vi "上位机.vi"() -> ()   [LabVIEW 2017]
uses:
  HslCommunication.dll
panel:
  in  "启动时读取数据":bool
  out "总时间 2":u32 format="%.0fms"
  out "PLC单次读写时间":u32 format="%.0fms"
  out "数值":i32
  out "Q14.6 备用":bool
  out "Q10.0 三色灯红":bool
  out "Q10.1 三色灯黄":bool
  out "Q10.2 三色灯绿":bool
  out "Q10.6 循环停止指示":bool
  out "Q10.7 原点指示":bool
  out "Q11.0 备用":bool
  out "Q14.0 工位1选择检测型腔":bool
  out "Q14.1 工位1选择检测水道":bool
  out "Q14.2 工位1选择检测回油道":bool
  out "Q14.7 辊道电机变频器启动":bool
  out "Q15.0 试漏启动":bool
  out "Q15.1 试漏频道0#":bool
  out "Q15.2 试漏频道1#":bool
  out "Q15.3 试漏频道2#":bool
  out "Q15.4 试漏频道3#":bool
  out "Q15.5 备用":bool
  out "Q15.6 备用":bool
  out "Q15.7 备用":bool
  out "Q14.3 工位1型腔泄压":bool
  out "Q14.4 工位1水道泄压":bool
  out "Q14.5 工位1选择回油道泄压":bool
  out "Q10.3 三色灯蜂鸣":bool
  out "Q10.4 故障复位指示":bool
  out "Q10.5 循环启动指示":bool
  out "Q11.1 备用":bool
  out "I10.0 机器人电源反馈":bool
  out "I10.1 伺服电源反馈":bool
  out "I10.2 输送电源反馈":bool
  out "I10.3 备用":bool
  out "I10.4 备用":bool
  out "I10.5 备用":bool
  out "I10.6 备用":bool
  out "I10.7 备用":bool
  out "I11.0 系统上电":bool
  out "I11.1 急停":bool
  out "I11.2 故障复位":bool
  out "I11.3 备用":bool
  out "I11.4 备用":bool
  out "I12.0 1#萃盘物料上升检测":bool
  out "I12.2 1#萃盘上料皮带检测1":bool
  out "I12.4 1#萃盘下料皮带检测1":bool
  out "I12.6 备用":bool
  out "I12.7 备用":bool
  out "I13.0 2#萃盘物料上升检测":bool
  out "I13.1 2#萃盘物料倾斜检测":bool
  out "I13.2 2#萃盘上料皮带检测1":bool
  out "I13.3 2#萃盘上料皮带检测2":bool
  out "I13.4 2#萃盘下料皮带检测1":bool
  out "I13.5 2#萃盘下料皮带检测2":bool
  out "I13.6 备用":bool
  out "I13.7 备用":bool
  out "I14.0 1#X轴气缸原位":bool
  out "I14.1 1#X轴气缸工作位":bool
  out "I14.2 1#Z轴气缸原位":bool
  out "I14.3  1#Z轴气缸工作位":bool
  out "I14.4  2#X轴气缸原位":bool
  out "I14.5  2#X轴气缸工作位":bool
  out "I14.6  2#Z轴气缸原位":bool
  out "I14.7  2#Z轴气缸工作位":bool
  out "I15.0  热熔升降原位":bool
  out "I15.1  热熔升降工作位":bool
  out "I15.2  烧录升降原位":bool
  out "I15.3  烧录升降工作位":bool
  out "I15.4  备用":bool
  out "I15.5  备用":bool
  out "I15.6  备用":bool
  out "I15.7  备用":bool
  out "I12.1 1#萃盘物料倾斜检测":bool
  out "I12.3 1#萃盘上料皮带检测2":bool
  out "I12.5 1#萃盘下料皮带检测2":bool
  in  "缩回按钮":bool
  in  "伸出按钮":bool
  in  "缩回按钮 2":bool
  in  "伸出按钮 2":bool
  in  "缩回按钮 3":bool
  in  "伸出按钮 3":bool
  in  "缩回按钮 4":bool
  in  "伸出按钮 4":bool
  in  "缩回按钮 5":bool
  in  "伸出按钮 5":bool
  in  "缩回按钮 6":bool
  in  "伸出按钮 6":bool
  in  "缩回按钮 7":bool
  in  "伸出按钮 7":bool
  in  "缩回按钮 8":bool
  in  "伸出按钮 8":bool
  in  "缩回按钮 9":bool
  in  "伸出按钮 9":bool
  in  "缩回按钮 10":bool
  in  "伸出按钮 10":bool
  in  "缩回按钮 11":bool
  in  "伸出按钮 11":bool
  in  "缩回按钮 12":bool
  in  "伸出按钮 12":bool
  out "M210.0 自动模式":bool
  out "通讯状态":bool
  out "模式选择":i32(ring) items=["单机模式", "联机模式"]
  out "产品信号":i32(ring) items=["CS-18", ""]
  out "设备状态":i32(ring) items=["准备OK"]
  out "当前报警代码":i32 format="%x"
  out "当前故障代码":i32 format="%x"
  out "1轴转速":dbl
  out "1轴转速 2":dbl
  out "1轴转速 3":dbl
  in  "1#轴位置5":dbl
  in  "1#轴位置3":dbl
  in  "1#轴位置4":dbl
  in  "1#轴位置1":dbl
  in  "1#轴位置2":dbl
  in  "2#轴位置5":dbl
  in  "2#轴位置3":dbl
  in  "2#轴位置4":dbl
  in  "2#轴位置1":dbl
  in  "2#轴位置2":dbl
  out "连接成功 2":bool
  # "IO布尔读取DB1.4"
  # "布尔写入DB1.0"
  # "IO布尔读取DB1.20"
  # "浮点数写入DB1.284"
  # "浮点数读取DB1.160"
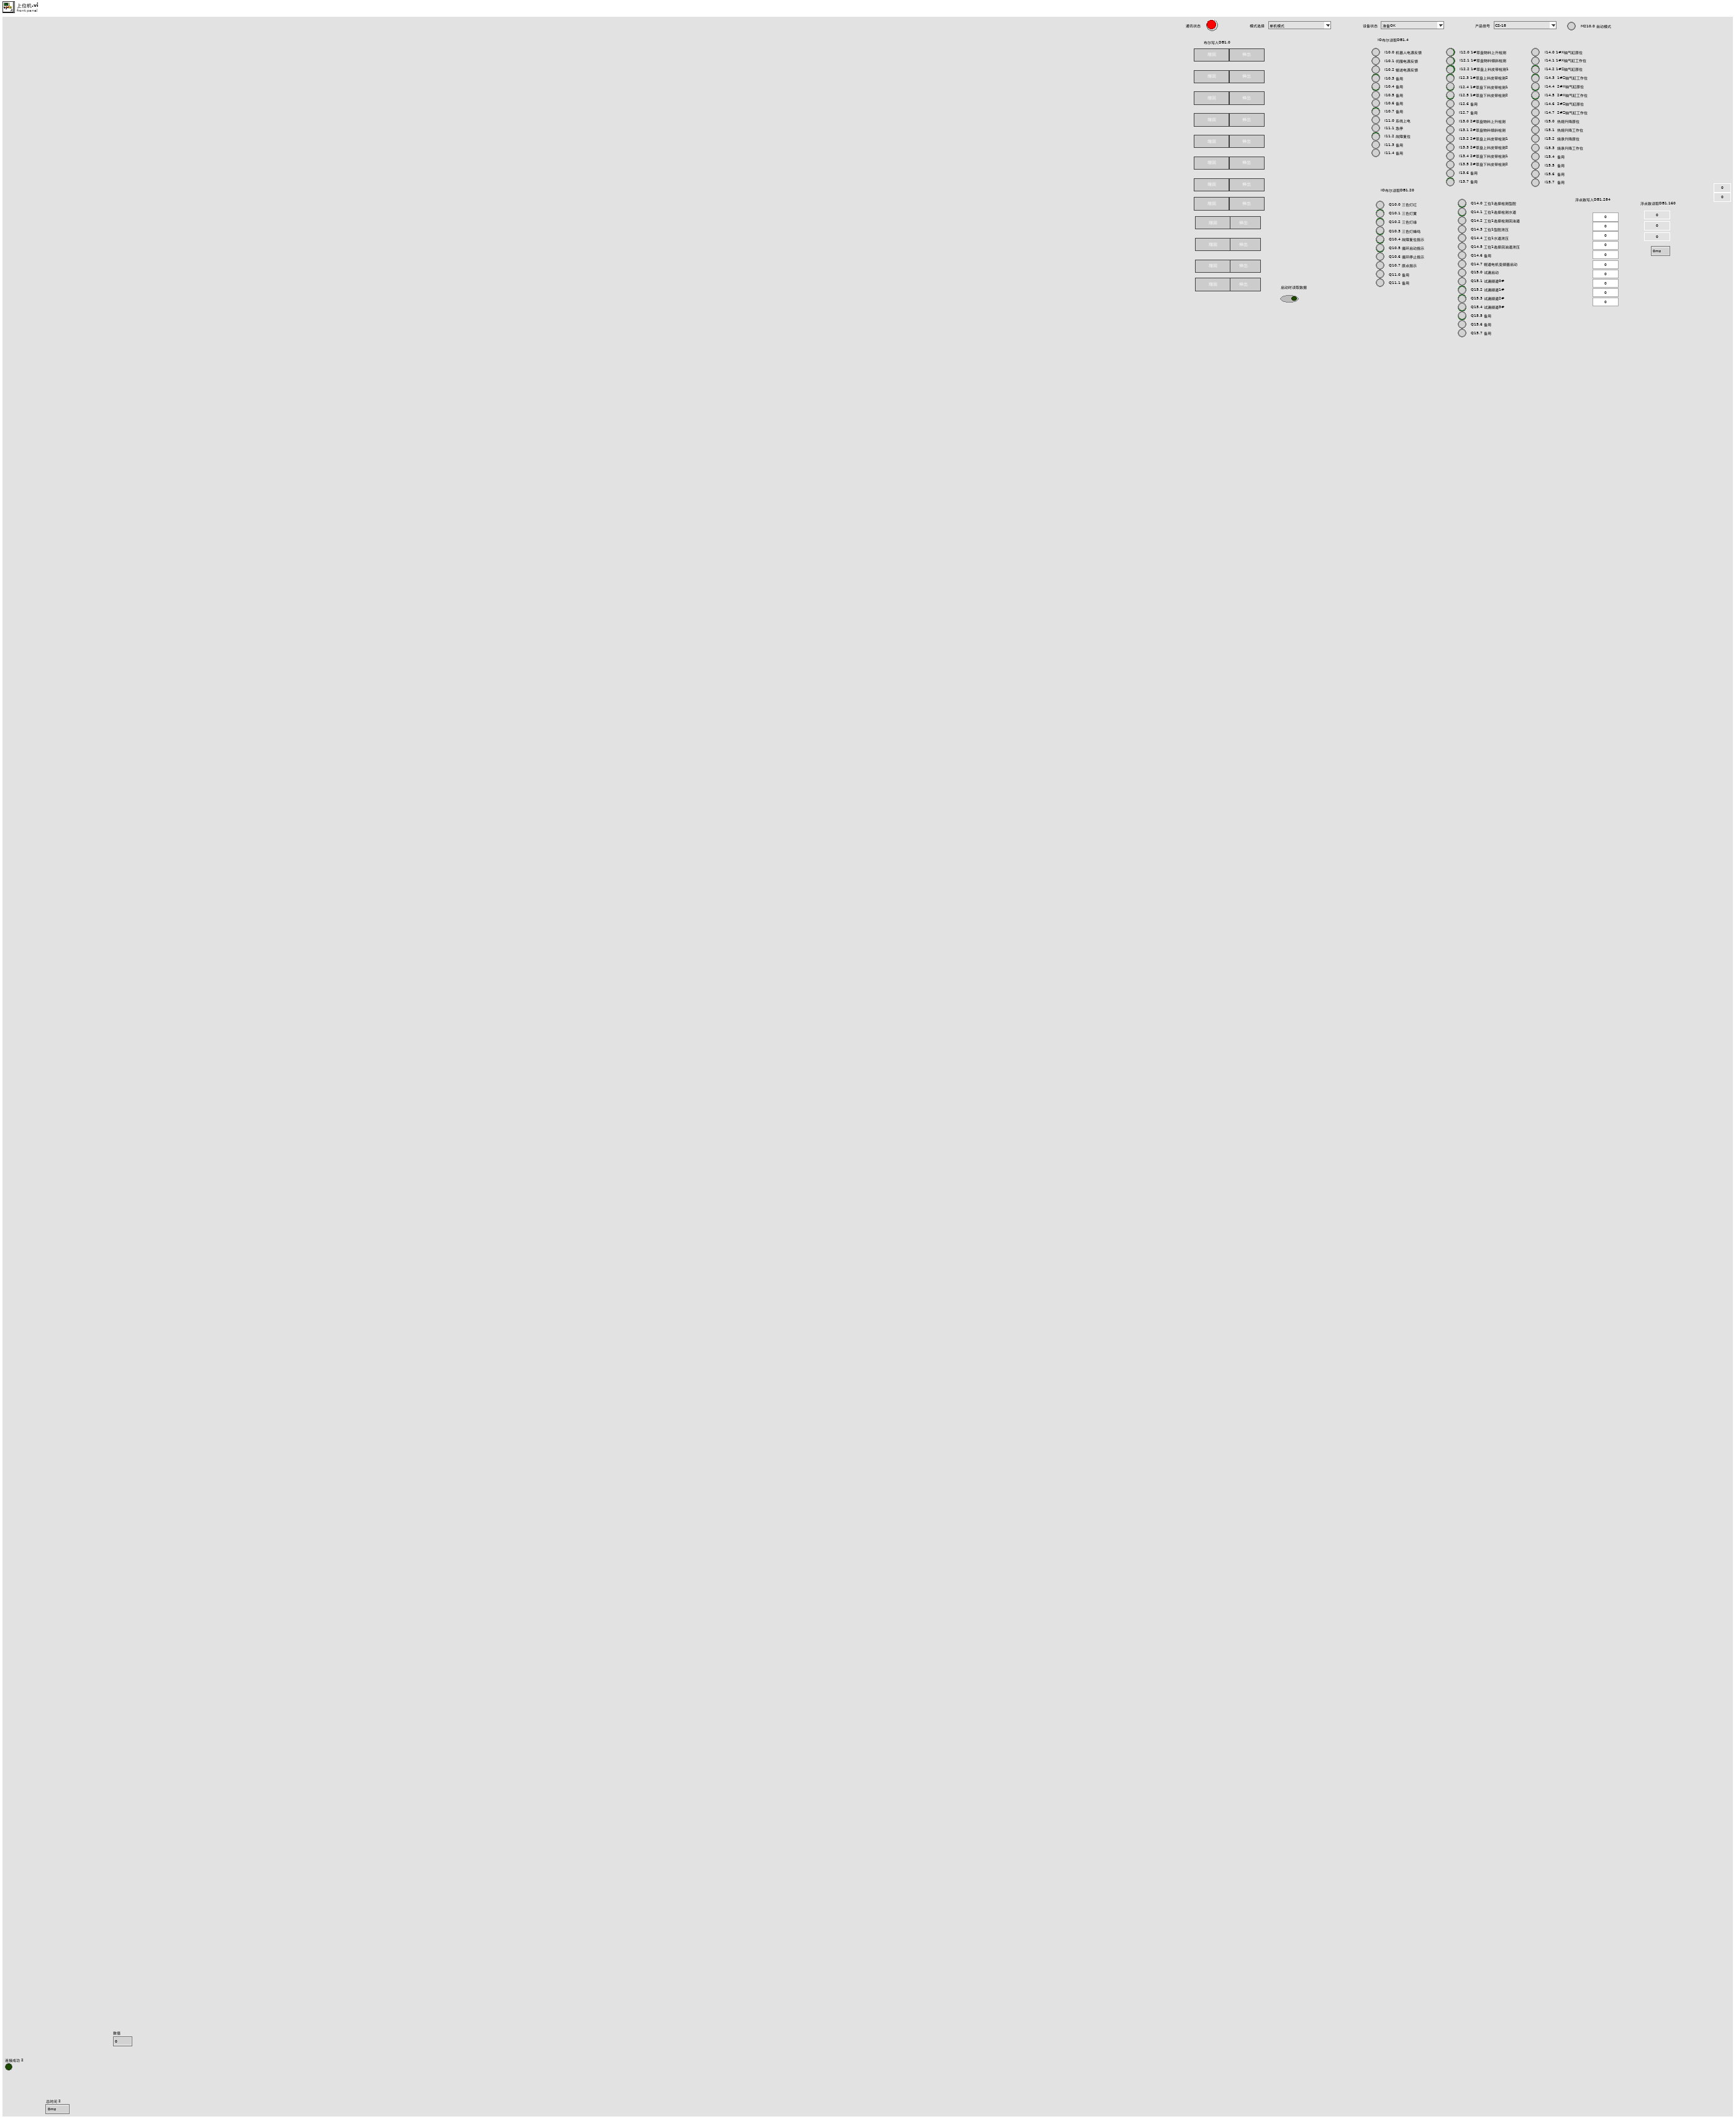
[diagram p1: front panel]
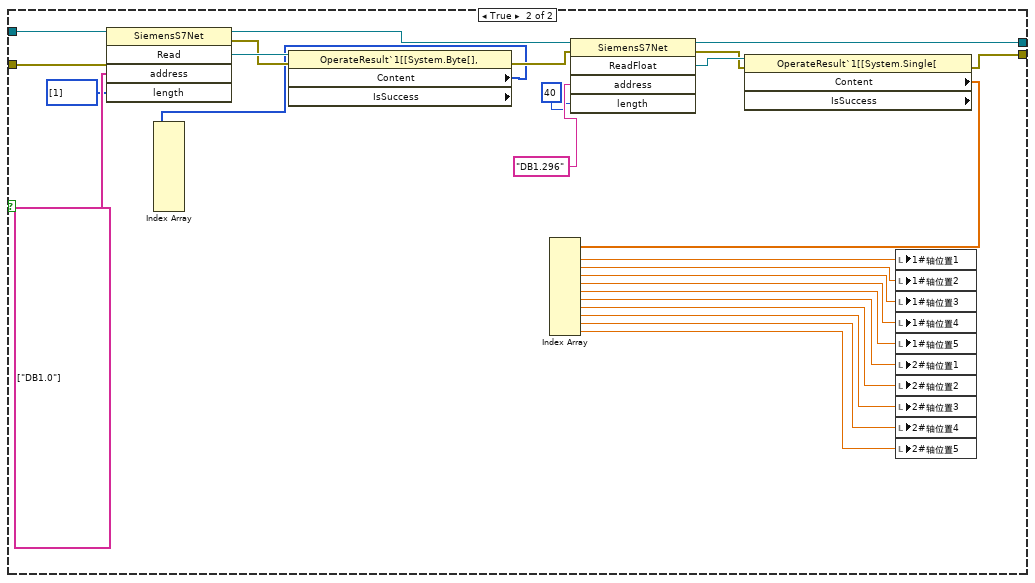
[diagram p3: hidden frame]
diagram:
  n1 = while {
    tunnel: [w5] -> _
    tunnel: [w2] -> _
    stop <- FALSE stop-if-true
    n2 = flat-sequence {
      tunnel: [w9] -> w8
      tunnel: w8 -> [w21]
      tunnel: [w21] -> w7
      tunnel: [w13] -> w5
      tunnel: [w12] -> w3
      tunnel: w7 -> [w314]
      tunnel: w3 -> [w313]
      tunnel: [w313] -> w2
      frame #0 {
        n3 = Tick Count (ms)() -> (millisecond timer value=w9:u32)
      }
      frame #1 {
        w17 = 4 items=["S1200"=1, "S300"=2, "S400"=3, "S1500"=4, "S200Smart"=5] ("siemens")
        n4 = constructor class="SiemensS7Net"("siemens"=w17, "ipAddress"="192.168.10.10") -> (reference out=w15:refnum<k24>, error out=w14:errorcluster)  [unwired: 3 in, 3 out]
        n5 = invoke class="SiemensS7Net" method="ConnectServer"(reference=w15, error in=w14) -> (reference out=w20:refnum<k24>, error out=w10:errorcluster, "ConnectServer"=w18:refnum<k24>)  [unwired: 1 in]
        n6 = property class="OperateResult"(reference=w18, error in=w10) -> (error out=w19:errorcluster, "IsSuccess"=w11:bool)  [unwired: 1 out]
        "连接成功 2" <- w11
        "通讯状态" <- w11
        n7 = case shown="真" w11 {
          tunnel: w20 -> [w23 w29]
          tunnel: w19 -> [w22 w28]
          tunnel: [w23 w25] -> w13
          tunnel: [w22 w24] -> w12
          frame False {
          }
          frame True {
            n8 = flat-sequence {
              tunnel: w28 -> [w40]
              tunnel: w29 -> [w41]
              tunnel: [w39] -> w36
              tunnel: [w38] -> w35
              tunnel: [w42] -> w34
              tunnel: w36 -> [w76]
              tunnel: w35 -> [w75]
              tunnel: [w74] -> w33
              tunnel: [w73] -> w32
              tunnel: [w72] -> w31
              tunnel: w34 -> [w72]
              tunnel: [w71] -> w30
              tunnel: [w311] -> w26
              tunnel: [w312] -> w27
              tunnel: w33 -> [w312]
              tunnel: w32 -> [w311]
              tunnel: w31 -> [w309]
              tunnel: w30 -> [w307]
              frame #0 {
                n9 = local read "启动时读取数据"() -> (w37:bool)
                n10 = case shown="假" w37 {
                  tunnel: w41 -> [w44 w70]
                  tunnel: w40 -> [w43 w69]
                  tunnel: [w44 w64] -> w39
                  tunnel: [w43 w59] -> w38
                  frame False {
                  }
                  frame True {
                    n11 = invoke class="SiemensS7Net" method="Read"(reference=w70, error in=w69, "address"=string[] ["DB1.0"], "length"=u16[] [1]) -> (reference out=w65:refnum<k24>, error out=w66:errorcluster, "Read"=w68:refnum<k24>)  [unwired: 1 in, 2 out]
                    n12 = property class="OperateResult`1[[System.Byte[]," props=["Content", "IsSuccess"](reference=w68, error in=w66) -> (error out=w62:errorcluster, "Content"=w46:u8[])  [unwired: 2 out]
                    n13 = Index Array(array=w46) -> ()  [unwired: 9 in, 9 out]
                    n14 = invoke class="SiemensS7Net" method="ReadFloat"(reference=w65, error in=w62, "address"="DB1.296", "length"=u16 40) -> (reference out=w64:refnum<k24>, error out=w60:errorcluster, "ReadFloat"=w61:refnum<k24>)  [unwired: 1 in, 2 out]
                    n15 = property class="OperateResult`1[[System.Single[" props=["Content", "IsSuccess"](reference=w61, error in=w60) -> (error out=w59:errorcluster, "Content"=w58:sgl[])  [unwired: 2 out]
                    n16 = Index Array(array=w58) -> (element #1=w57:sgl, element #2=w56:sgl, element #3=w55:sgl, element #4=w54:sgl, element #5=w53:sgl, element #6=w52:sgl, element #7=w51:sgl, element #8=w50:sgl, element #9=w49:sgl, element #10=w48:sgl)  [unwired: 10 in]
                    n17 = local write "1#轴位置1"(w57) -> ()
                    n18 = local write "1#轴位置2"(w56) -> ()
                    n19 = local write "1#轴位置3"(w55) -> ()
                    n20 = local write "1#轴位置4"(w54) -> ()
                    n21 = local write "1#轴位置5"(w53) -> ()
                    n22 = local write "2#轴位置1"(w52) -> ()
                    n23 = local write "2#轴位置2"(w51) -> ()
                    n24 = local write "2#轴位置3"(w50) -> ()
                    n25 = local write "2#轴位置4"(w49) -> ()
                    n26 = local write "2#轴位置5"(w48) -> ()
                  }
                }
                n27 = Tick Count (ms)() -> (millisecond timer value=w42:u32)
              }
              frame #1 {
                w71 = 1 ("读写次数 2")
                n28 = for {
                  N: w71 -> [_]
                  shift-right: [w293] -> w74
                  shift-left: w76 -> [w297]
                  shift-right: [w290] -> w73
                  shift-left: w75 -> [w296]
                  i -> [w304]
                  w224 = "%"
                  w237 = " PCS"
                  w209 = u16 16
                  # "读取主界面，伺服故障和报警代码"
                  # "读取轴1到轴8的速度，当前位置，以及JOG当前轴位置"
                  # "布尔数组监控"
                  n29 = local write "启动时读取数据"(FALSE ("布尔")) -> ()
                  n30 = local write "通讯状态"(FALSE ("通讯状态")) -> ()
                  n31 = Build Array("缩回按钮", "伸出按钮", "缩回按钮 2", "伸出按钮 2", "缩回按钮 3", "伸出按钮 3", "缩回按钮 4", "伸出按钮 4", "缩回按钮 5", "伸出按钮 5", "缩回按钮 6", "伸出按钮 6", "缩回按钮 7", "伸出按钮 7", "缩回按钮 8", "伸出按钮 8", "缩回按钮 9", "伸出按钮 9", "缩回按钮 10", "伸出按钮 10", "缩回按钮 11", "伸出按钮 11", "缩回按钮 12", "伸出按钮 12") -> (w298:bool[])
                  n32 = invoke class="SiemensS7Net" method="Write"(reference=w297, error in=w296, "address"="DB1.0", "values"=w298) -> (reference out=w264:refnum<k24>, error out=w263:errorcluster)  [unwired: 1 in, 3 out]
                  n33 = invoke class="SiemensS7Net" method="ReadInt32"(reference=w264, error in=w263, "address"="DB1.36", "length"=u16 31) -> (reference out=w236:refnum<k24>, error out=w234:errorcluster, "ReadInt32"=w260:refnum<k24>)  [unwired: 1 in, 2 out]
                  n34 = property class="OperateResult`1[[System.Int32[]" props=["Content", "IsSuccess"](reference=w260) -> ("Content"=w259:i32[])  [unwired: 1 in, 3 out]
                  n35 = Index Array(array=w259) -> (element #1=→"模式选择":i32, element #2=→"设备状态":i32, element #3=→"产品信号":i32, element #4=w255:i32, element #5=w254:i32, element #6=w253:i32, element #7=w252:i32, element #8=w251:i32, element #9=w250:i32, element #10=w249:i32, element #11=w248:i32, element #12=w247:i32, element #13=→"当前报警代码":i32, element #14=→"当前故障代码":i32)  [unwired: 14 in]
                  n36 = Number To Decimal String(number=w255) -> (decimal integer string=w244:string)  [unwired: 1 in]
                  n37 = Number To Decimal String(number=w254) -> (decimal integer string=w243:string)  [unwired: 1 in]
                  n38 = Number To Decimal String(number=w253) -> (decimal integer string=w242:string)  [unwired: 1 in]
                  n39 = Number To Decimal String(number=w252) -> (decimal integer string=w241:string)  [unwired: 1 in]
                  n40 = Number To Decimal String(number=w251) -> (decimal integer string=w240:string)  [unwired: 1 in]
                  n41 = Number To Decimal String(number=w250) -> (decimal integer string=w239:string)  [unwired: 1 in]
                  n42 = Number To Decimal String(number=w249) -> (decimal integer string=w238:string)  [unwired: 1 in]
                  n43 = Number To Decimal String(number=w248) -> (decimal integer string=w226:string)  [unwired: 1 in]
                  n44 = Number To Decimal String(number=w247) -> (decimal integer string=w225:string)  [unwired: 1 in]
                  n45 = Concatenate Strings(w225, w224) -> ()  [unwired: 1 out]
                  n46 = Concatenate Strings(w244, w237) -> ()  [unwired: 1 out]
                  n47 = Concatenate Strings(w243, w237) -> ()  [unwired: 1 out]
                  n48 = Concatenate Strings(w242, w237) -> ()  [unwired: 1 out]
                  n49 = Concatenate Strings(w241, w237) -> ()  [unwired: 1 out]
                  n50 = Concatenate Strings(w240, w237) -> ()  [unwired: 1 out]
                  n51 = Concatenate Strings(w239, w237) -> ()  [unwired: 1 out]
                  n52 = Concatenate Strings(w238, w237) -> ()  [unwired: 1 out]
                  n53 = Concatenate Strings(w226, w224) -> ()  [unwired: 1 out]
                  n54 = invoke class="SiemensS7Net" method="ReadFloat"(reference=w236, error in=w234, "address"="DB1.160", "length"=u16 17) -> (reference out=w223:refnum<k24>, error out=w227:errorcluster, "ReadFloat"=w232:refnum<k24>)  [unwired: 1 in, 2 out]
                  n55 = property class="OperateResult`1[[System.Single[" props=["Content", "IsSuccess"](reference=w232, error in=w227) -> (error out=w210:errorcluster, "Content"=w231:sgl[])  [unwired: 2 out]
                  n56 = Index Array(array=w231) -> (element #1=→"1轴转速":sgl, element #2=→"1轴转速 2":sgl, element #3=→"1轴转速 3":sgl)  [unwired: 3 in]
                  n57 = Build Array("1#轴位置1", "1#轴位置2", "1#轴位置3", "1#轴位置4", "1#轴位置5", "2#轴位置1", "2#轴位置2", "2#轴位置3", "2#轴位置4", "2#轴位置5") -> (w211:dbl[])
                  n58 = invoke class="SiemensS7Net" method="Write"(reference=w223, error in=w210, "address"="DB1.284", "values"=w211) -> (reference out=w79:refnum<k24>, error out=w78:errorcluster)  [unwired: 1 in, 3 out]
                  n59 = Build Array(w209, w209) -> (w302:u16[])
                  n60 = invoke class="SiemensS7Net" method="Read"(reference=w79, error in=w78, "address"=string[] ["DB1.4", "DB1.20"], "length"=w302) -> (reference out=w295:refnum<k24>, "Read"=w303:refnum<k24>)  [unwired: 1 in, 3 out]
                  n61 = property class="OperateResult`1[[System.Byte[]," props=["Content", "IsSuccess"](reference=w303) -> (error out=w292:errorcluster, "Content"=w152:u8[])  [unwired: 1 in, 2 out]
                  n62 = Index Array(array=w152) -> (element #1=w208:u8, element #2=w198:u8, element #3=w192:u8, element #4=w191:u8, element #5=w190:u8, element #6=w189:u8, element #7=w187:u8, element #8=w185:u8, element #17=w142:u8, element #18=w141:u8, element #19=w140:u8, element #20=w139:u8, element #21=w138:u8, element #22=w137:u8, element #23=w136:u8, element #24=w135:u8)  [unwired: 24 in, 8 out]
                  n63 = Number To Boolean Array(number=w208) -> (Boolean array=w207:bool[])
                  n64 = Number To Boolean Array(number=w141) -> (Boolean array=w179:bool[])
                  n65 = Number To Boolean Array(number=w142) -> (Boolean array=w184:bool[])
                  n66 = Number To Boolean Array(number=w198) -> (Boolean array=w197:bool[])
                  n67 = Index Array(array=w207) -> (element #1=→"I10.0 机器人电源反馈":bool, element #2=→"I10.1 伺服电源反馈":bool, element #3=→"I10.2 输送电源反馈":bool, element #4=→"I10.3 备用":bool, element #5=→"I10.4 备用":bool, element #6=→"I10.5 备用":bool, element #7=→"I10.6 备用":bool, element #8=→"I10.7 备用":bool)  [unwired: 8 in]
                  n68 = Index Array(array=w197) -> ()  [unwired: 8 in, 8 out]
                  n69 = Index Array(array=w184) -> (element #1=→"Q10.0 三色灯红":bool, element #2=→"Q10.1 三色灯黄":bool, element #3=→"Q10.2 三色灯绿":bool, element #4=→"Q10.3 三色灯蜂鸣":bool, element #5=→"Q10.4 故障复位指示":bool, element #6=→"Q10.5 循环启动指示":bool, element #7=→"Q10.6 循环停止指示":bool, element #8=→"Q10.7 原点指示":bool)  [unwired: 8 in]
                  n70 = Index Array(array=w179) -> (element #1=→"Q11.0 备用":bool, element #2=→"Q11.1 备用":bool)  [unwired: 8 in, 6 out]
                  n71 = Number To Boolean Array(number=w192) -> (Boolean array=w196:bool[])
                  n72 = Number To Boolean Array(number=w139) -> (Boolean array=w182:bool[])
                  n73 = Number To Boolean Array(number=w191) -> (Boolean array=w195:bool[])
                  n74 = Number To Boolean Array(number=w140) -> (Boolean array=w183:bool[])
                  n75 = Index Array(array=w195) -> (element #1=→"I13.0 2#萃盘物料上升检测":bool, element #2=→"I13.1 2#萃盘物料倾斜检测":bool, element #3=→"I13.2 2#萃盘上料皮带检测1":bool, element #4=→"I13.3 2#萃盘上料皮带检测2":bool, element #5=→"I13.4 2#萃盘下料皮带检测1":bool, element #6=→"I13.5 2#萃盘下料皮带检测2":bool, element #7=→"I13.6 备用":bool, element #8=→"I13.7 备用":bool)  [unwired: 8 in]
                  n76 = Index Array(array=w182) -> ()  [unwired: 8 in, 8 out]
                  n77 = Index Array(array=w183) -> ()  [unwired: 8 in, 8 out]
                  n78 = Index Array(array=w196) -> (element #1=→"I12.0 1#萃盘物料上升检测":bool, element #2=→"I12.1 1#萃盘物料倾斜检测":bool, element #3=→"I12.2 1#萃盘上料皮带检测1":bool, element #4=→"I12.3 1#萃盘上料皮带检测2":bool, element #5=→"I12.4 1#萃盘下料皮带检测1":bool, element #6=→"I12.5 1#萃盘下料皮带检测2":bool, element #7=→"I12.6 备用":bool, element #8=→"I12.7 备用":bool)  [unwired: 8 in]
                  n79 = Number To Boolean Array(number=w190) -> (Boolean array=w194:bool[])
                  n80 = Number To Boolean Array(number=w137) -> (Boolean array=w180:bool[])
                  n81 = Number To Boolean Array(number=w189) -> (Boolean array=w193:bool[])
                  n82 = Number To Boolean Array(number=w138) -> (Boolean array=w181:bool[])
                  n83 = Index Array(array=w193) -> (element #1=→"I15.0  热熔升降原位":bool, element #2=→"I15.1  热熔升降工作位":bool, element #3=→"I15.2  烧录升降原位":bool, element #4=→"I15.3  烧录升降工作位":bool, element #5=→"I15.4  备用":bool, element #6=→"I15.5  备用":bool, element #7=→"I15.6  备用":bool, element #8=→"I15.7  备用":bool)  [unwired: 8 in]
                  n84 = Index Array(array=w194) -> (element #1=→"I14.0 1#X轴气缸原位":bool, element #2=→"I14.1 1#X轴气缸工作位":bool, element #3=→"I14.2 1#Z轴气缸原位":bool, element #4=→"I14.3  1#Z轴气缸工作位":bool, element #5=→"I14.4  2#X轴气缸原位":bool, element #6=→"I14.5  2#X轴气缸工作位":bool, element #7=→"I14.6  2#Z轴气缸原位":bool, element #8=→"I14.7  2#Z轴气缸工作位":bool)  [unwired: 8 in]
                  n85 = Index Array(array=w180) -> (element #1=→"Q15.0 试漏启动":bool, element #2=→"Q15.1 试漏频道0#":bool, element #3=→"Q15.2 试漏频道1#":bool, element #4=→"Q15.3 试漏频道2#":bool, element #5=→"Q15.4 试漏频道3#":bool, element #6=→"Q15.5 备用":bool, element #7=→"Q15.6 备用":bool, element #8=→"Q15.7 备用":bool)  [unwired: 8 in]
                  n86 = Index Array(array=w181) -> (element #1=→"Q14.0 工位1选择检测型腔":bool, element #2=→"Q14.1 工位1选择检测水道":bool, element #3=→"Q14.2 工位1选择检测回油道":bool, element #4=→"Q14.3 工位1型腔泄压":bool, element #5=→"Q14.4 工位1水道泄压":bool, element #6=→"Q14.5 工位1选择回油道泄压":bool, element #7=→"Q14.6 备用":bool, element #8=→"Q14.7 辊道电机变频器启动":bool)  [unwired: 8 in]
                  n87 = Build Array(u16 1 ("元素")) -> (w287:u16[])
                  n88 = invoke class="SiemensS7Net" method="Read"(reference=w295, error in=w292, "address"=string[] ["I100"], "length"=w287) -> (reference out=w293:refnum<k24>, error out=w291:errorcluster, "Read"=w294:refnum<k24>)  [unwired: 1 in, 2 out]
                  n89 = Number To Boolean Array(number=w187) -> (Boolean array=w186:bool[])
                  n90 = Number To Boolean Array(number=w185) -> (Boolean array=w188:bool[])
                  n91 = property class="OperateResult`1[[System.Byte[]," props=["Content", "IsSuccess"](reference=w294, error in=w291) -> (error out=w290:errorcluster)  [unwired: 3 out]
                  n92 = Number To Boolean Array(number=w135) -> (Boolean array=w93:bool[])
                  n93 = Number To Boolean Array(number=w136) -> (Boolean array=w94:bool[])
                  n94 = Index Array(array=w93) -> ()  [unwired: 8 in, 8 out]
                  n95 = Index Array(array=w94) -> ()  [unwired: 8 in, 8 out]
                  n96 = Index Array(array=w186) -> ()  [unwired: 8 in, 8 out]
                  n97 = Index Array(array=w188) -> ()  [unwired: 8 in, 8 out]
                  n98 = Index Array(array=w152) -> (element #9=w134:u8, element #10=w133:u8, element #11=w132:u8, element #12=w131:u8, element #13=w130:u8, element #14=w129:u8, element #15=w128:u8, element #16=w127:u8, element #25=w86:u8, element #26=w85:u8, element #27=w84:u8, element #28=w83:u8, element #29=w82:u8, element #30=w81:u8)  [unwired: 34 in, 20 out]
                  n99 = Number To Boolean Array(number=w85) -> (Boolean array=w92:bool[])
                  n100 = Number To Boolean Array(number=w86) -> (Boolean array=w91:bool[])
                  n101 = Index Array(array=w92) -> ()  [unwired: 8 in, 8 out]
                  n102 = Index Array(array=w91) -> ()  [unwired: 8 in, 8 out]
                  n103 = Number To Boolean Array(number=w134) -> (Boolean array=w151:bool[])
                  n104 = Number To Boolean Array(number=w133) -> (Boolean array=w150:bool[])
                  n105 = Index Array(array=w151) -> ()  [unwired: 8 in, 8 out]
                  n106 = Index Array(array=w150) -> ()  [unwired: 8 in, 8 out]
                  n107 = Number To Boolean Array(number=w83) -> (Boolean array=w89:bool[])
                  n108 = Number To Boolean Array(number=w84) -> (Boolean array=w90:bool[])
                  n109 = Number To Boolean Array(number=w132) -> (Boolean array=w148:bool[])
                  n110 = Number To Boolean Array(number=w131) -> (Boolean array=w149:bool[])
                  n111 = Index Array(array=w89) -> ()  [unwired: 8 in, 8 out]
                  n112 = Index Array(array=w90) -> ()  [unwired: 8 in, 8 out]
                  n113 = Index Array(array=w148) -> ()  [unwired: 8 in, 8 out]
                  n114 = Index Array(array=w149) -> ()  [unwired: 8 in, 8 out]
                  n115 = Number To Boolean Array(number=w81) -> (Boolean array=w88:bool[])
                  n116 = Number To Boolean Array(number=w82) -> (Boolean array=w87:bool[])
                  n117 = Number To Boolean Array(number=w130) -> (Boolean array=w147:bool[])
                  n118 = Number To Boolean Array(number=w129) -> (Boolean array=w146:bool[])
                  n119 = Index Array(array=w88) -> ()  [unwired: 8 in, 8 out]
                  n120 = Index Array(array=w87) -> ()  [unwired: 8 in, 8 out]
                  n121 = Index Array(array=w147) -> ()  [unwired: 8 in, 8 out]
                  n122 = Index Array(array=w146) -> ()  [unwired: 8 in, 8 out]
                  n123 = Number To Boolean Array(number=w128) -> (Boolean array=w144:bool[])
                  n124 = Number To Boolean Array(number=w127) -> (Boolean array=w145:bool[])
                  n125 = Index Array(array=w144) -> ()  [unwired: 8 in, 8 out]
                  n126 = Index Array(array=w145) -> ()  [unwired: 8 in, 8 out]
                  "数值" <- w304
                }
              }
              frame #2 {
                n127 = Tick Count (ms)() -> (millisecond timer value=w310:u32)
                n128 = Subtract(x=w310, y=w309) -> (x-y=w308:u32)
                n129 = Divide(x=w308, y=w307) -> (x/y=w306:dbl)
                n130 = To Unsigned Long Integer(number=w306) -> (unsigned 32bit integer=→"PLC单次读写时间":u32)
              }
            }
            n131 = invoke class="SiemensS7Net" method="ConnectClose"(reference=w27, error in=w26) -> (reference out=w25:refnum<k24>, error out=w24:errorcluster)  [unwired: 1 in, 1 out]
          }
        }
      }
      frame #2 {
        n132 = Tick Count (ms)() -> (millisecond timer value=w315:u32)
        n133 = Subtract(x=w315, y=w314) -> (x-y=→"总时间 2":u32)
      }
    }
    n134 = Wait (ms)(milliseconds to wait=u32 10 ("等待时间（毫秒）")) -> ()  [unwired: 1 out]
  }
  n135 = local write "启动时读取数据"(TRUE ("启动时读取数据")) -> ()
